vi "Hysteresis-Correct_1_piezo.vi"(9 "Hyst curve":dbl[](array[numeric]), 11 "Image In":dbl[][](array[numeric])) -> (3 "Image Out":dbl[][](array[numeric]))   [LabVIEW 2016]
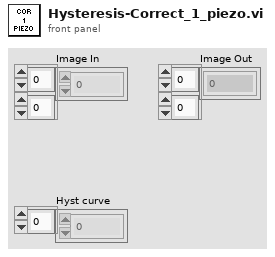
[diagram p1: front panel]
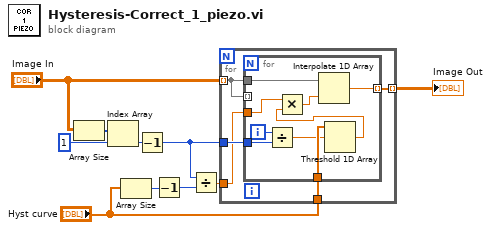
[diagram p0: block diagram]
diagram:
  n1 = Array Size(array="Image In") -> (size(s)=w10:i32[])
  n2 = Index Array(array=w10, index=1) -> (element=w8:i32)
  n3 = Array Size(array="Hyst curve") -> (size(s)=w5:i32)
  n4 = Decrement(x=w8) -> (x-1=w7:i32)
  n5 = Decrement(x=w5) -> (x-1=w3:i32)
  n6 = Divide(x=w7, y=w3) -> (x/y=w6:dbl)
  n7 = for {
    tunnel: "Image In" -> [w12] mode=indexing
    tunnel: w7 -> [w15]
    tunnel: "Hyst curve" -> [w14]
    tunnel: [w13] -> w2 mode=indexing
    tunnel: w6 -> [w11]
    n8 = for {
      tunnel: w15 -> [w23]
      tunnel: w14 -> [w22]
      tunnel: w12 -> [w21]
      tunnel: [w20] -> w13 mode=indexing
      tunnel: w12 -> [_] mode=indexing
      tunnel: w11 -> [w17]
      i -> [w24]
      n9 = Divide(x=w24, y=w23) -> (x/y=w19:dbl)
      n10 = Threshold 1D Array(2:w19, 3:w22) -> (0:w18:dbl)  [unwired: 1 in]
      n11 = Multiply(x=w17, y=w18) -> (x*y=w16:dbl)
      n12 = Interpolate 1D Array(1:w16, 2:w21) -> (0:w20:dbl)
    }
  }
  "Image Out" <- w2
